vi "Power Accuracy Initialize Test.vi"(7 "Files Found?":bool=TRUE, 8 "error in (no error)":errorcluster, 9 "Instruments to Use":T15, 10 "Seq Count":u32, 11 "Test Parameters In":T2={"Stimulus"={"Power Start"=38, "Power Stop"=46, "Frequency Type"=enum."Band Edges", "Frequency Points"=[], "TX 1 Frequency (MHz)"={"Min"=0.0, "Max"=0.0}, "TX 2 Frequency (MHz)"={"Min"=0.0, "Max"=0.0}, "RX Frequency (MHz)"={"Min"=0.0, "Max"=0.0}, "Pad Model Number"="", "Pad Serial Number"="", "Pad Values"=[]}, "Measurement"={"DUT Port"=enum."Port 1", "Direction"=0}, "Display"={"Power"={"Min"=0, "Max"=0}, "Tolerance"={"Min"=0.0, "Max"=0.0}}, "Limit"={"Tolerance"=0.35}, "Calibration"={"Calibrated?"=FALSE}} {"Measurement"."Direction" items=["Reverse", "Forward", "Auxiliary"]}) -> (0 "error out":errorcluster, 1 "Test Parameters Out":T2={"Stimulus"={"Power Start"=38, "Power Stop"=46, "Frequency Type"=enum."Band Edges", "Frequency Points"=[], "TX 1 Frequency (MHz)"={"Min"=0.0, "Max"=0.0}, "TX 2 Frequency (MHz)"={"Min"=0.0, "Max"=0.0}, "RX Frequency (MHz)"={"Min"=0.0, "Max"=0.0}, "Pad Model Number"="", "Pad Serial Number"="", "Pad Values"=[]}, "Measurement"={"DUT Port"=enum."Port 1", "Direction"=0}, "Display"={"Power"={"Min"=0, "Max"=0}, "Tolerance"={"Min"=0.0, "Max"=0.0}}, "Limit"={"Tolerance"=0.35}, "Calibration"={"Calibrated?"=FALSE}} {"Measurement"."Direction" items=["Reverse", "Forward", "Auxiliary"]}, 2 "Next Action":string, 3 "Instrument IDs":T1, 4 "Driver Refs":T13, 5 "TestSetDef":T10={"General"={"ID"=0, "Model"="", "Dual Port?"=FALSE, "Options"="", "Options"={"E"=FALSE, "K"=FALSE, "H"=FALSE, "W"=FALSE, "F"=FALSE}, "Cal File"=path ""}, "Receiver"={"Fstart, MHz"=0.0, "Fstop MHz"=0.0, "Fstep MHz"=0.0, "IF, MHz"=0.0}, "RX Band"={"Fstart, MHz"=0.0, "Fstop MHz"=0.0}, "TX 1"={"Fstart, MHz"=0.0, "Fstop MHz"=0.0, "Pmax, dBm"=0.0, "Pstep, dB"=0.0}, "TX 2"={"Fstart, MHz"=0.0, "Fstop MHz"=0.0, "Pmax, dBm"=0.0, "Pstep, dB"=0.0}, "Low-side?"=TRUE}, 6 "Instrument In-Cal?":bool)   [LabVIEW 2011]
uses:
  TypeDefs/Power Accuracy Test Parameters.ctl
  TypeDefs/Power Accuracy Stimulus Parameters.ctl
  TypeDefs/Power Accuracy Measurement Parameters.ctl
  SI.LIB/PIM.LIB/HW IO/DUTport.ctl
  SI.LIB/PIM.LIB/HW IO/MeasMode.ctl
  TypeDefs/Power Accuracy Display Parameters.ctl
  TypeDefs/Power Accuracy Limit Parameters.ctl
  TypeDefs/Power Accuracy Calibration State.ctl
  server/database/Stations/Instruments/Instrument Record.ctl
  drivers/PIM/PIM Driver Ref.ctl
  drivers/PWM/PWM Driver Ref.ctl
  SI.LIB/PIM.LIB/HW IO/Test Set Definition.ctl
  drivers/PWM/PWM Command.ctl
  drivers/PIM/PIM Command.ctl
  OpenG.LIB/array/array.llb/Remove Duplicates from 1D Array (DBL)__ogtk.vi
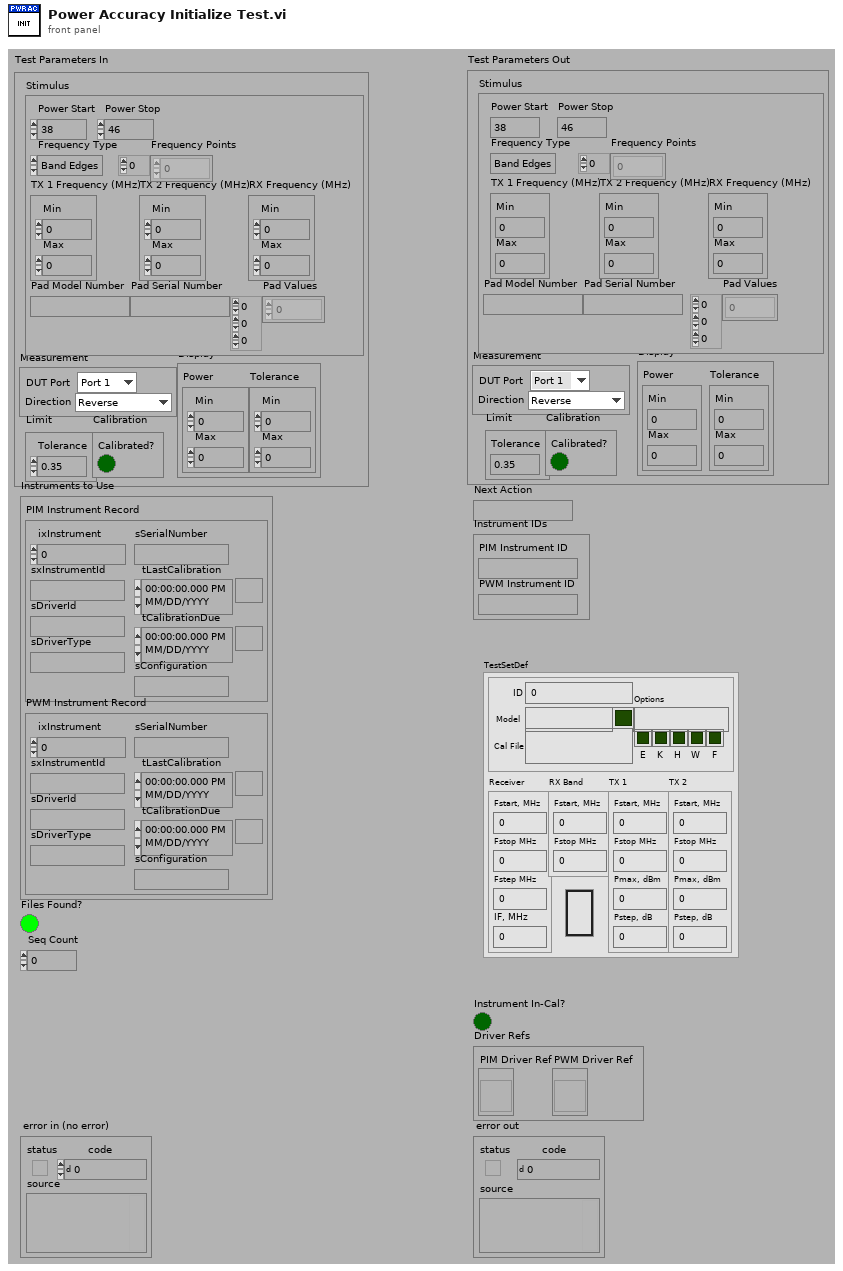
[diagram p1: front panel]
types:
  T1 = cluster{"PIM Instrument ID":string, "PWM Instrument ID":string}
  T2 = typedef "Power Accuracy Test Parameters.ctl" = cluster{"Stimulus":T3, "Measurement":T4, "Display":T7, "Limit":T8, "Calibration":T9}
  T3 = typedef "Power Accuracy Stimulus Parameters.ctl" = cluster{"Power Start":i32, "Power Stop":i32, "Frequency Type":enum16{"Band Edges", "Custom"}, "Frequency Points":dbl[], "TX 1 Frequency (MHz)":cluster{"Min":dbl, "Max":dbl}, "TX 2 Frequency (MHz)":cluster{"Min":dbl, "Max":dbl}, "RX Frequency (MHz)":cluster{"Min":dbl, "Max":dbl}, "Pad Model Number":string, "Pad Serial Number":string, "Pad Values":dbl[][][]}
  T4 = typedef "Power Accuracy Measurement Parameters.ctl" = cluster{"DUT Port":T5, "Direction":T6}
  T5 = typedef "DUTport.ctl" = enum16{"Port 1", "Port 2"}
  T6 = typedef "MeasMode.ctl" = u16
  T7 = typedef "Power Accuracy Display Parameters.ctl" = cluster{"Power":cluster{"Min":i32, "Max":i32}, "Tolerance":cluster{"Min":dbl, "Max":dbl}}
  T8 = typedef "Power Accuracy Limit Parameters.ctl" = cluster{"Tolerance":dbl}
  T9 = typedef "Power Accuracy Calibration State.ctl" = cluster{"Calibrated?":bool}
  T10 = typedef "Test Set Definition.ctl" = cluster{"General":cluster{"ID":u32, "Model":string, "Dual Port?":bool, "Options":string, "Options":cluster{"E":bool, "K":bool, "H":bool, "W":bool, "F":bool}, "Cal File":path}, "Receiver":cluster{"Fstart, MHz":dbl, "Fstop MHz":dbl, "Fstep MHz":dbl, "IF, MHz":dbl}, "RX Band":cluster{"Fstart, MHz":dbl, "Fstop MHz":dbl}, "TX 1":cluster{"Fstart, MHz":dbl, "Fstop MHz":dbl, "Pmax, dBm":dbl, "Pstep, dB":dbl}, "TX 2":cluster{"Fstart, MHz":dbl, "Fstop MHz":dbl, "Pmax, dBm":dbl, "Pstep, dB":dbl}, "Low-side?":bool}
  T11 = typedef "PIM Driver Ref.ctl" = refnum<vi>
  T12 = typedef "PWM Driver Ref.ctl" = refnum<vi>
  T13 = cluster{"PIM Driver Ref":T11, "PWM Driver Ref":T12}
  T14 = typedef "Instrument Record.ctl" = cluster{"ixInstrument":i32, "sxInstrumentId":string, "sDriverId":string, "sDriverType":string, "sSerialNumber":string, "tLastCalibration":timestamp, "tCalibrationDue":timestamp, "sConfiguration":string}
  T15 = cluster{"PIM Instrument Record":T14, "PWM Instrument Record":T14}
  T16 = typedef "PWM Command.ctl" = enum16{"LOAD", "INITIALIZE", "PRESET", "GET STIMULUS", "SET STIMULUS", "MEASURE", "RELEASE", "UNLOAD", "GET CALIBRATION", "CALIBRATE"}
  T17 = typedef "PIM Command.ctl" = enum16{"LOAD", "KEEP ALIVE", "VALIDATE", "INITIALIZE", "PRESET", "GET CALIBRATION", "SET STIMULUS", "TOGGLE TX POWER", "SET TX ON", "SET TX OFF", "MEASURE", "UNLOAD"}
  T18 = typedef "PWM Normalization State.ctl" = bool
  T19 = typedef "PIM Stimulus.ctl" = cluster{"Carrier Frequencies":cluster{"C1 Freq, MHz":dbl, "C2 Freq, MHz":dbl}, "Carrier Powers":cluster{"C1 Power,dBm":dbl, "C2 Power, dBm":dbl}, "Measurement Parameters":T20, "Measurement Setup":cluster{"Meas Type":enum32{"Time", "Frequency"}, "TXStep":T24}}
  T20 = typedef "PIM Cmd Params.ctl" = cluster{"IM Order":T21, "Averaging":T22, "Direction":T6, "Enable ALC?":bool, "Enable SingleIM?":bool, "Display Units":T23, "VA Hold?":bool, "DUT PORT":T5}
  T21 = typedef "IMOrder.ctl" = u8
  T22 = typedef "HW Averaging.ctl" = u16
  T23 = typedef "display_unit_format.ctl" = enum16{"dBm", "dBc"}
  T24 = typedef "PIM Sweep Step Size.ctl" = u16
  T25 = cluster{"duplicate driver ref":T11, "dup Drv Refnum":T12}
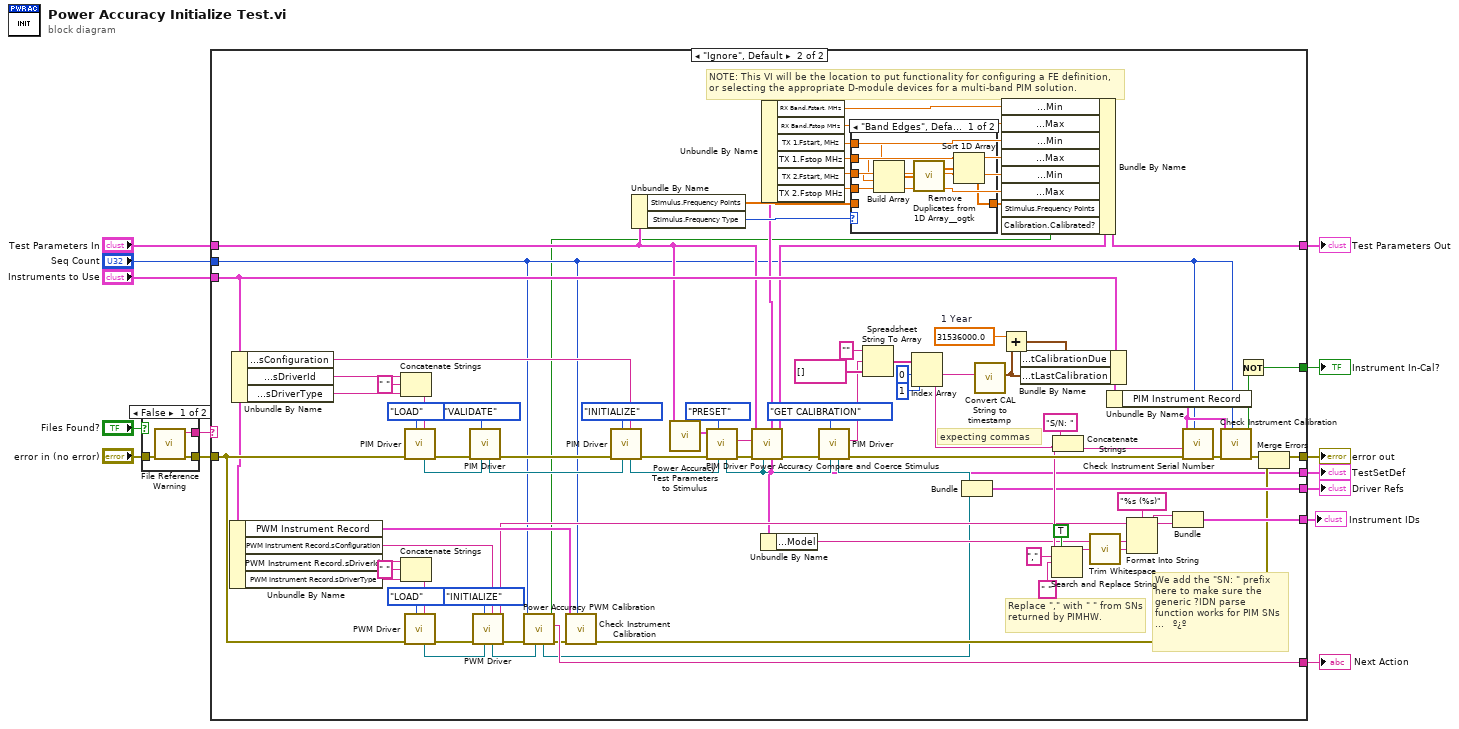
[diagram p0: block diagram]
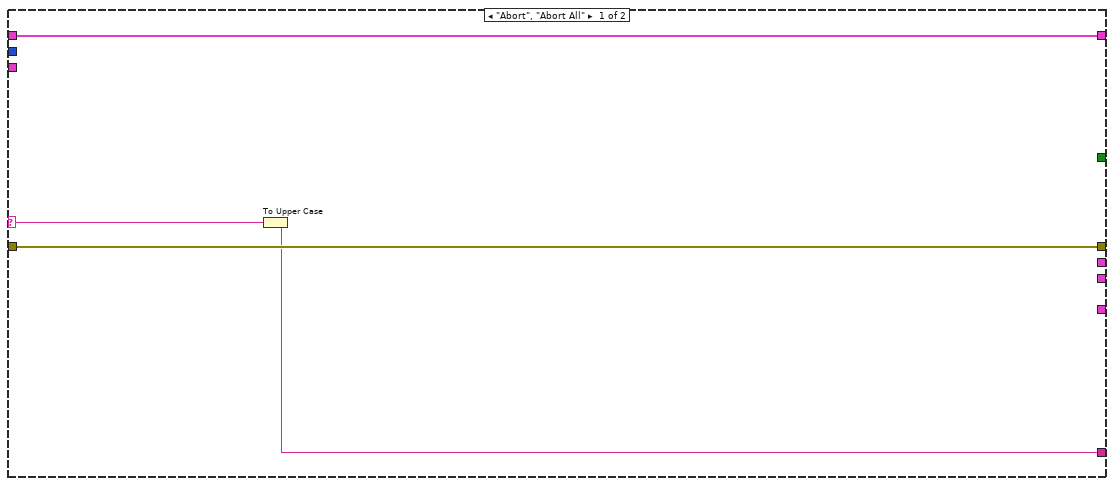
[diagram p2: hidden frame]
diagram:
  n1 = case shown="False" "Files Found?" {
    tunnel: "error in (no error)" -> [w17 w18]
    tunnel: [w16 w18] -> w3
    tunnel: [w15 _] -> w6
    frame False {
      n2 = call "File Reference Warning.vi"("error in (no error)"=w17) -> ("error out"=w16:errorcluster, "Command"=w15:string)  [unwired: 9 out]
    }
    frame True {
    }
  }
  n3 = case shown="\"Ignore\", Default" w6 {
    selector: w6 -> [w20 _]
    tunnel: [_ w36] -> w14
    tunnel: [_ w91] -> w13
    tunnel: [w22 w43] -> w12
    tunnel: "Test Parameters In" -> [w19 w42]
    tunnel: [w19 w39] -> w10
    tunnel: w3 -> [w22 w78]
    tunnel: "Instruments to Use" -> [_ w66]
    tunnel: "Seq Count" -> [_ w27]
    tunnel: [w21 w26] -> w5
    tunnel: [_ w52] -> w2
    tunnel: [_ w46] -> w1
    frame "Abort", "Abort All" {
      n4 = To Upper Case(1:w20) -> (0:w21:string)
    }
    frame "Ignore", Default {
      w95 = 31536000.0  # 1 Year
      # "expecting commas"
      # "Replace \",\" with \" \" from SNs returned by PIMHW."
      # "NOTE: This VI will be the location to put functionality for configuring a FE definition, or selecting the appropriate D-module devices for a multi-band PIM solution."
      # "We add the \"SN: \" prefix here to make sure the generic ?IDN parse function works for PIM SNs ...   º¿º"
      n5 = Unbundle By Name(w66) -> ("PWM Instrument Record"=w54:T14, "PWM Instrument Record.sConfiguration"=w65:string, "PWM Instrument Record.sDriverId"=w59:string, "PWM Instrument Record.sDriverType"=w58:string)
      n6 = Unbundle By Name(w66) -> ("PIM Instrument Record.sConfiguration"=w108:string, "PIM Instrument Record.sDriverId"=w62:string, "PIM Instrument Record.sDriverType"=w61:string)
      n7 = Concatenate Strings(w62, " " ("string"), w61) -> (w60:string)
      n8 = Concatenate Strings(w59, " " ("string"), w58) -> (w57:string)
      n9 = call "PIM Driver.vi"("PIM Driver Name/Configuration"=w60, "PIM Command"=PIM_Command."LOAD", "error in (no error)"=w78) -> ("error out"=w76:errorcluster, "duplicate driver ref"=w74:T11)  [unwired: 2 in, 5 out]
      n10 = call "PWM Driver.vi"("PWM Configuration (\"\")"=w57, "PWM Command"=PWM_Command."LOAD" ("DMM Command"), "error in (no error)"=w78) -> ("error out"=w68:errorcluster, "dup Drv Refnum"=w67:T12)  [unwired: 5 in, 2 out]
      n11 = call "PIM Driver.vi"("Driver Ref (null)"=w74, "PIM Command"=PIM_Command."VALIDATE", "error in (no error)"=w76) -> ("error out"=w75:errorcluster, "duplicate driver ref"=w73:T11)  [unwired: 2 in, 5 out]
      n12 = call "PWM Driver.vi"("PWM Configuration (\"\")"=w65, "Drv Refnum"=w67, "PWM Command"=PWM_Command."INITIALIZE" ("DMM Command"), "error in (no error)"=w68) -> ("error out"=w29:errorcluster, "Variant Output"=w51:string, "dup Drv Refnum"=w28:T12)  [unwired: 4 in, 1 out]
      n13 = call "Power Accuracy PWM Calibration.vi"("Drv Refnum"=w28, "error in (no error)"=w29, "Seq Count"=w27) -> ("error out"=w24:errorcluster, "Next Action"=w26:string, "Calibrated?"=w23:T18, "dup Drv Refnum"=w25:T12)  [unwired: 5 in]
      n14 = call "Check Instrument Calibration.vi"("Seq Count"=w27, "error in (no error)"=w24, "Instrument Record"=w54) -> ("error out"=w45:errorcluster)  [unwired: 1 in, 7 out]
      n15 = call "PIM Driver.vi"("PIM Driver Name/Configuration"=w108, "Driver Ref (null)"=w73, "PIM Command"=PIM_Command."INITIALIZE", "error in (no error)"=w75) -> ("error out"=w90:errorcluster, "duplicate driver ref"=w72:T11)  [unwired: 1 in, 5 out]
      n16 = Unbundle By Name(w42) -> ("Stimulus.Frequency Points"=w41:dbl[], "Stimulus.Frequency Type"=w37:enum16{"Band Edges", "Custom"})
      n17 = call "Power Accuracy Test Parameters to Stimulus.vi"("Power Accuracy Test Parameters"=w42) -> ("PIM Measurement Stimulus"=w85:T19)  [unwired: 10 out]
      n18 = call "PIM Driver.vi"("Driver Ref (null)"=w72, "PIM Command"=PIM_Command."PRESET", "error in (no error)"=w90, "Stimulus"=w85) -> ("error out"=w96:errorcluster, "Variant Output"=w97:string, "duplicate driver ref"=w71:T11)  [unwired: 1 in, 4 out]
      n19 = call "Power Accuracy Compare and Coerce Stimulus.vi"("Driver Ref (null)"=w71, "error in (no error)"=w96, "Flat TestSetDef Params"=w97, "PV Test Parameters"=w42) -> ("error out"=w89:errorcluster, "Corrected Test Params"=w40:T2, "TestSetDef"=w36:T10)  [unwired: 5 out]
      n20 = Unbundle By Name(w36) -> ("General.Model"=w49:string)
      n21 = Unbundle By Name(w36) -> ("RX Band.Fstart, MHz"=w34:dbl, "RX Band.Fstop MHz"=w35:dbl, "TX 1.Fstart, MHz"=w30:dbl, "TX 1.Fstop MHz"=w31:dbl, "TX 2.Fstart, MHz"=w32:dbl, "TX 2.Fstop MHz"=w33:dbl)
      n22 = call "PIM Driver.vi"("Driver Ref (null)"=w71, "PIM Command"=PIM_Command."GET CALIBRATION", "error in (no error)"=w89) -> ("error out"=w86:errorcluster, "Variant Output"=w87:string, "duplicate driver ref"=w53:T11)  [unwired: 2 in, 4 out]
      n23 = case shown="\"Band Edges\", Default" w37 {
        tunnel: w41 -> [_ w117]
        tunnel: [w114 w117] -> w38
        tunnel: w33 -> [w112 _]
        tunnel: w32 -> [w111 _]
        tunnel: w31 -> [w110 _]
        tunnel: w30 -> [w113 _]
        frame "Band Edges", Default {
          n24 = Build Array(w113, w110, w111, w112) -> (w116:dbl[])
          n25 = call-poly "Remove Duplicates from 1D Array__ogtk.vi"("Input Array"=w116) -> ("Output Array"=w115:dbl[])  [unwired: 1 out]
          n26 = Sort 1D Array(array=w115) -> (sorted array=w114:dbl[])
        }
        frame "Custom" {
        }
      }
      n27 = Spreadsheet String To Array(format string="", spreadsheet string=w87, array type (2D Dbl)=string[] []) -> (array=w107:string[])  [unwired: 1 out]
      n28 = Index Array(array=w107, index #1=0 ("index"), index #2=1 ("index")) -> (element #1=w102:string, element #2=w80:string)
      n29 = Bundle("duplicate driver ref"=w53, "dup Drv Refnum"=w25) -> (w52:T25)  [unwired: 1 in]
      n30 = call "Convert CAL String to timestamp.vi"("abbreviated date string"=w102) -> ("time stamp"=w94:timestamp)  [unwired: 10 out]
      n31 = Add(x=w95, y=w94) -> (x+y=w93:timestamp)
      n32 = Bundle By Name(cluster=w40, "Stimulus.RX Frequency (MHz).Min"=w34, "Stimulus.RX Frequency (MHz).Max"=w35, "Stimulus.TX 1 Frequency (MHz).Min"=w30, "Stimulus.TX 1 Frequency (MHz).Max"=w31, "Stimulus.TX 2 Frequency (MHz).Min"=w32, "Stimulus.TX 2 Frequency (MHz).Max"=w33, "Stimulus.Frequency Points"=w38, "Calibration.Calibrated?"=w23) -> (w39:T2)
      n33 = Bundle By Name(cluster=w66, "PIM Instrument Record.tCalibrationDue"=w93, "PIM Instrument Record.tLastCalibration"=w94) -> (w56:T15)
      n34 = Search and Replace String(replace all?=TRUE ("replace all? (F)"), input string=w80, search string="," ("delimiter (Tab)"), replace string=" " ("replace string (\"\")")) -> (result string=w81:string)  [unwired: 1 in, 6 out]
      n35 = Concatenate Strings("S/N: ", w80) -> (w99:string)
      n36 = call <vilib>:"Trim Whitespace.vi"("string"=w81) -> ("trimmed string"=w48:string)  [unwired: 1 in]
      n37 = Unbundle By Name(w56) -> ("PIM Instrument Record"=w55:T14)
      n38 = Format Into String(format string="%s (%s)", w49, w48) -> (resulting string=w47:string)  [unwired: 2 in, 1 out]
      n39 = Bundle(w47, "Variant Output"=w51) -> (w46:cluster{string, "Variant Output":string})  [unwired: 1 in]
      n40 = call "Check Instrument Serial Number.vi"("Seq Count"=w27, "error in (no error)"=w86, "Instrument IDN String (\"\")"=w99, "Instrument Record"=w55) -> ("error out"=w101:errorcluster)  [unwired: 7 out]
      n41 = call "Check Instrument Calibration.vi"("Seq Count"=w27, "error in (no error)"=w101, "Instrument Record"=w55) -> ("error out"=w44:errorcluster, "Cal Expired?"=w92:bool)  [unwired: 7 out]
      n42 = Not(x=w92) -> (.not. x?=w91:bool)
      n43 = Merge Errors(w44, w45) -> (w43:errorcluster)
    }
  }
  "Driver Refs" <- w2
  "error out" <- w12
  "TestSetDef" <- w14
  "Instrument In-Cal?" <- w13
  "Test Parameters Out" <- w10
  "Next Action" <- w5
  "Instrument IDs" <- w1
